vi "Generater.TestLauncher.vi"() -> ()   [LabVIEW 2019, in "Generator.lvclass"]
uses:
  Generator.lvclass
  typedefs/AO.Channel--Cluster--Array.ctl
  typedefs/AO.Channel--Cluster.ctl
  typedefs/AO.Channel.Function--Enum.ctl
  typedefs/REF.Channel--Cluster--Array.ctl
  typedefs/REF.Channel--Cluster.ctl
  typedefs/Sampling--Cluster.ctl
  typedefs/Sweep.Configuration--Cluster.ctl
  typedefs/Sweep.Channel--Cluster--Array.ctl
  typedefs/Sweep.Channel--Cluster.ctl
  typedefs/Sweep.Pattern--Enum.ctl
  typedefs/Generator.Command--enum.ctl
  typedefs/Generator.Sweep Status--enum.ctl
  <userlib>/LevyLab/Debug/Attribute.Debug/DebugBehavior.ctl
  C:/Program Files/National Instruments/LabVIEW 2019/vi.lib/JKI/JKI SMO/SMO/SMO.lvclass
  <vilib>/JKI/JKI SMO/SMO/SMO.lvclass/SMO.ctl
  <vilib>/JKI/JKI SMO/SMO/Typedefs/SMOState --Enum.ctl
  <vilib>/JKI/JKI SMO/SMO/Private/ReftoDVR--SMO.vi
  <vilib>/JKI/JKI SMO/SMO/SMO.lvclass
  <userlib>/LevyLab/Debug/Debug.lvlib
  <userlib>/LevyLab/Debug/Attribute.Debug/Attribute.Debug.lvclass
panel:
  in  "timeout":i32
  in  "Execute":bool
  out "sweep status":T1=enum."sweeping"
  out "Waveforms":waveform(dbl)[](graph)
  out "Waveform Chart":u32(graph)
  in  "command":T2=enum."stop"
  in  "Sweep Channels":T3 {"Channels"."Table" format="%#_1f"; "Channels"."Channel" min=1 max=128; "Channels"."Start" format="%#_6p"; "Channels"."End" format="%#_6p"}
  in  "Sampling":T7
  in  "REF Channels":T8
  in  "AO Channels":T10
  out "error out":errorcluster
  # "Close Panel to stop the SMO\n(press the \"X\")"
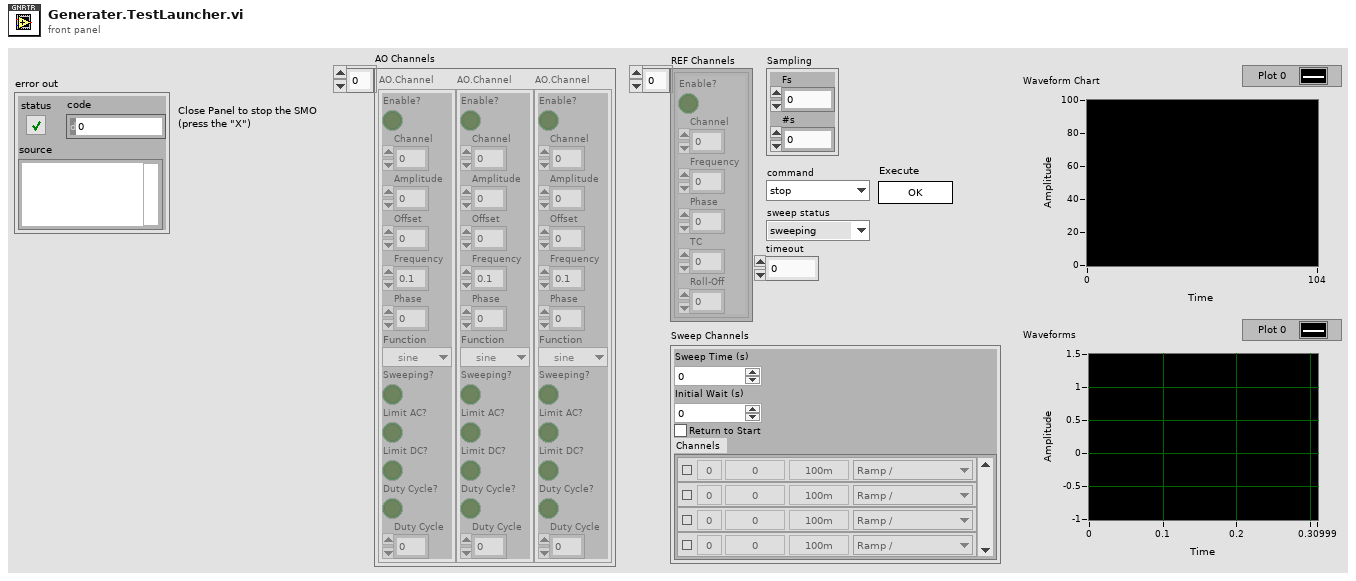
[diagram p1: front panel]
types:
  T1 = typedef "Generator.lvclass/Generator.Sweep Status--enum.ctl" = enum16{"idle", "initializing", "waiting", "sweeping", "stopping"}
  T2 = typedef "Generator.lvclass/Generator.Command--enum.ctl" = enum16{"start", "stop", "start sweep", "stop sweep"}
  T3 = typedef "Generator.lvclass/Sweep.Configuration--Cluster.ctl" = cluster{"Sweep Time (s)":dbl, "Initial Wait (s)":dbl, "Return to Start":bool, "Channels":T4}
  T4 = typedef "Generator.lvclass/Sweep.Channel--Cluster--Array.ctl" = T5[]
  T5 = typedef "Generator.lvclass/Sweep.Channel--Cluster.ctl" = cluster{"Enable?":bool, "Channel":u16, "Start":dbl, "End":dbl, "Pattern":T6, "Table":dbl[]}
  T6 = typedef "Generator.lvclass/Sweep.Pattern--Enum.ctl" = enum16{"Ramp /", "Ramp /\\", "Smooth Ramp _/", "Smooth Ramp _/\\_", "Table"}
  T7 = typedef "Generator.lvclass/Sampling--Cluster.ctl" = cluster{"Fs":dbl, "#s":dbl}
  T8 = typedef "Generator.lvclass/REF.Channel--Cluster--Array.ctl" = T9[]
  T9 = typedef "Generator.lvclass/REF.Channel--Cluster.ctl" = cluster{"Enable?":bool, "Channel":i32, "Frequency":dbl, "Phase":dbl, "TC":dbl, "Roll-Off":i32}
  T10 = typedef "Generator.lvclass/AO.Channel--Cluster--Array.ctl" = T11[]
  T11 = typedef "Generator.lvclass/AO.Channel--Cluster.ctl" = cluster{"Enable?":bool, "Channel":i32, "Amplitude":dbl, "Offset":dbl, "Frequency":dbl, "Phase":dbl, "Function":T12, "Sweeping?":bool, "Limit AC?":bool, "Limit DC?":bool, "Duty Cycle?":bool, "Duty Cycle":dbl}
  T12 = typedef "Generator.lvclass/AO.Channel.Function--Enum.ctl" = enum16{"sine", "square", "triangle", "saw"}
  T13 = typedef "Debug.lvlib/Attribute.Debug.lvclass/DebugBehavior.ctl" = enum16{"Normal", "Debug"}
  T14 = typedef "Generator.lvclass/PublicEvents--Cluster.ctl" = cluster{"Status":refnum<user-event>, "SweepStatus":refnum<user-event>, "AOChannels":refnum<user-event>, "Waveforms":refnum<user-event>}
  T15 = typedef "SMO.lvclass/Public Events.ctl" = cluster{"Error":refnum<user-event>, "State":refnum<user-event>, "Reserve State":refnum<user-event>}
  T16 = cluster{"Event Registration Refnum":refnum<event-registration>}
  T17 = typedef "SMO.lvclass/SMOState --Enum.ctl" = enum16{"unknown", "Created", "Started", "Stopped"}
  T18 = typedef "Generator.lvclass/Waveforms--Cluster.ctl" = cluster{"AO":waveform(dbl)[], "REF_X":waveform(dbl)[], "REF_Y":waveform(dbl)[]}
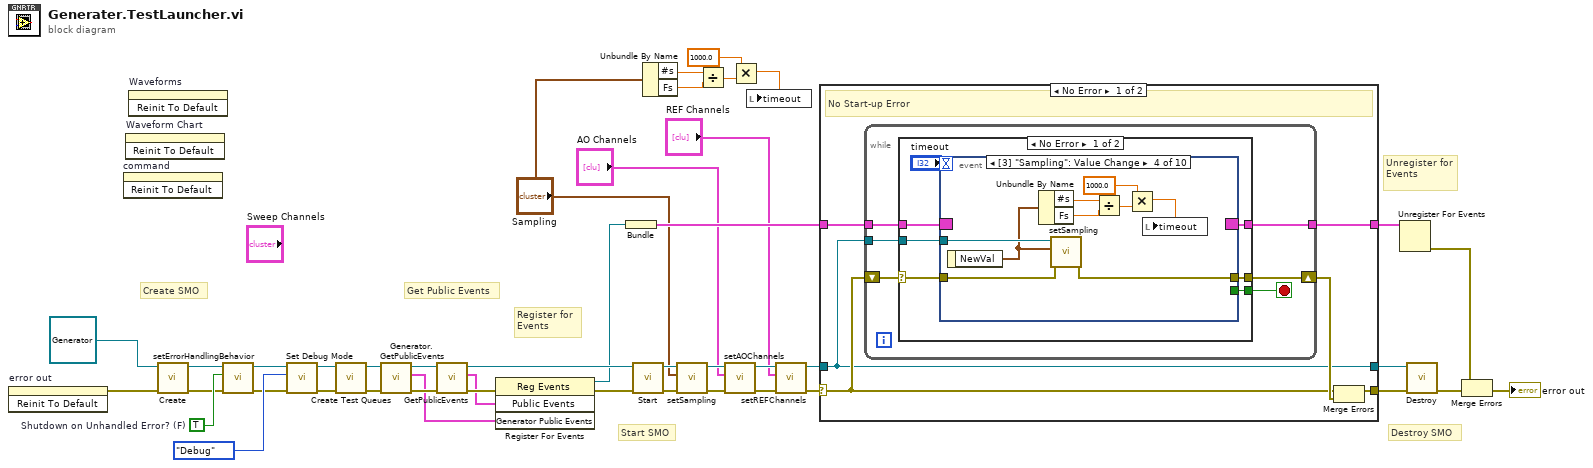
[diagram p0: block diagram]
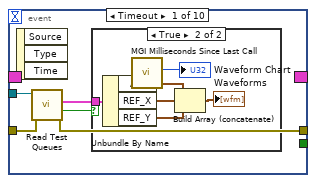
[diagram p2: hidden frame]
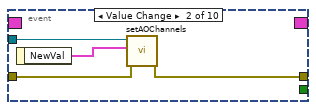
[diagram p4: hidden frame]
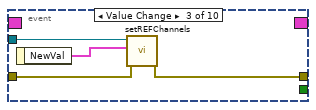
[diagram p5: hidden frame]
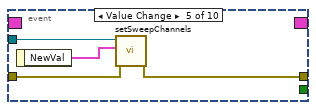
[diagram p6: hidden frame]
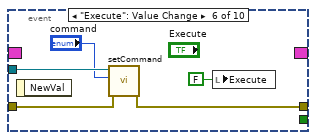
[diagram p7: hidden frame]
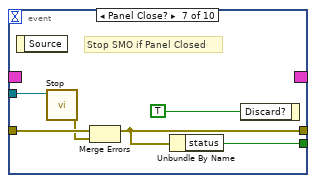
[diagram p8: hidden frame]
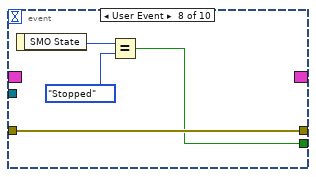
[diagram p9: hidden frame]
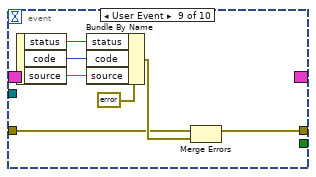
[diagram p10: hidden frame]
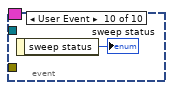
[diagram p11: hidden frame]
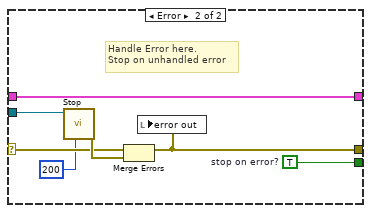
[diagram p12: hidden frame]
diagram:
  w40 = TRUE  # Shutdown on Unhandled Error? (F)
  # "Get Public Events"
  # "Start SMO"
  # "Destroy SMO"
  # "Create SMO"
  # "Unregister for Events"
  # "Register for Events"
  n1 = invoke on="error out" class="Clust (strict)" method="Reinit To Default"() -> (error out=w41:errorcluster)  [unwired: 3 in, 2 out]
  n2 = invoke on="command" class="Enum (strict)" method="Reinit To Default"() -> ()  [unwired: 3 in, 3 out]
  n3 = invoke on="Waveform Chart" class="WFChart (strict)" method="Reinit To Default"() -> ()  [unwired: 3 in, 3 out]
  n4 = invoke on="Waveforms" class="WFGraph (strict)" method="Reinit To Default"() -> ()  [unwired: 3 in, 3 out]
  n5 = call <vilib>:"Create.vi"("error in (no error)"=w41, "SMO"=refnum<class "Generator.lvclass"> refnum ("Generator.lvclass")) -> ("error out"=w39:errorcluster, "SMO out"=w38:refnum<class "Generator.lvclass">)  [unwired: 7 in, 1 out]
  n6 = call <vilib>:"setErrorHandlingBehavior.vi"("error in (no error)"=w39, "Shutdown on Unhandled Error? (F)"=w40, "SMO in"=w38) -> ("error out"=w24:errorcluster, "SMO out"=w25:refnum<class "Generator.lvclass">)  [unwired: 7 in]
  n7 = call <userlib>:"Set Debug Mode.vi"("error in (no error)"=w24, "Behavior"=DebugBehavior."Debug", "SMO"=w25) -> ("error out"=w11:errorcluster, "SMO out"=w23:refnum<class "Generator.lvclass">)  [unwired: 7 in]
  n8 = call "Create Test Queues.vi"("error in (no error)"=w11, "Generator in"=w23) -> ("error out"=w10:errorcluster, "Generator out"=w12:refnum<class "Generator.lvclass">)  [unwired: 8 in]
  n9 = call "Generator.GetPublicEvents.vi"("error in (no error)"=w10, "Generator"=w12) -> ("error out"=w9:errorcluster, "Generator Public Events"=w8:T14, "Generator out"=w7:refnum<class "Generator.lvclass">)  [unwired: 7 in]
  n10 = call <vilib>:"GetPublicEvents.vi"("error in (no error)"=w9, "SMO"=w7) -> ("error out"=w36:errorcluster, "Public Events"=w35:T15, "SMO out"=w42:refnum<class "Generator.lvclass">)  [unwired: 7 in]
  n11 = register-events(error in=w36, w35, w8) -> (reference out=w33:refnum<event-registration>, error out=w34:errorcluster)  [unwired: 1 in]
  n12 = Bundle("Event Registration Refnum"=w33) -> (w29:T16)  [unwired: 1 in]
  n13 = call <vilib>:"Start.vi"("error in (no error)"=w34, "SMO"=w42) -> ("error out"=w18:errorcluster, "SMO out"=w17:refnum<class "Generator.lvclass">)  [unwired: 8 in]
  n14 = Unbundle By Name("Sampling") -> ("#s"=w2:dbl, "Fs"=w3:dbl)
  n15 = call "setSampling.vi"("error in (no error)"=w18, "Sampling"="Sampling", "Generator in"=w17) -> ("error out"=w20:errorcluster, "Generator out"=w19:refnum<class "Generator.lvclass">)  [unwired: 7 in]
  n16 = Divide(x=w2, y=w3) -> (x/y=w4:dbl)
  n17 = call "setAOChannels.vi"("error in (no error)"=w20, "AO Channels"="AO Channels", "Generator in"=w19) -> ("error out"=w22:errorcluster, "Generator out"=w21:refnum<class "Generator.lvclass">)  [unwired: 7 in]
  n18 = Multiply(x=1000.0, y=w4) -> (x*y=w6:dbl)
  n19 = local write "timeout"(w6) -> ()
  n20 = call "setREFChannels.vi"("error in (no error)"=w22, "REF Channels"="REF Channels", "Generator in"=w21) -> ("error out"=w15:errorcluster, "Generator out"=w16:refnum<class "Generator.lvclass">)  [unwired: 7 in]
  n21 = case shown="No Error" w15 {
    selector: w15 -> [w45 w126]
    tunnel: [w49 w127] -> w28
    tunnel: w29 -> [w48 w127]
    tunnel: [w46 w126] -> w37
    tunnel: w16 -> [w44 w125]
    tunnel: [w44 w125] -> w43
    frame No Error {
      # "No Start-up Error"
      n22 = while {
        shift-right: [w54] -> w47
        shift-left: w45 -> [w50]
        tunnel: w48 -> [w53]
        tunnel: [w52] -> w49
        tunnel: w44 -> [w51]
        stop <- w55 stop-if-true
        n23 = case shown="No Error" w50 {
          selector: w50 -> [w57 w121]
          tunnel: [w62 w124] -> w55
          tunnel: [w61 w118] -> w54
          tunnel: w53 -> [w60 w123]
          tunnel: [w59 w123] -> w52
          tunnel: w51 -> [w58 w120]
          frame No Error {
            n24 = event shown="[3] \"Sampling\": Value Change" {
              selector: w60 -> [_ _ _ _ _ _ _ _ _ _]
              dyn-events: [_ _ _ _ _ _ _ _ _ _] -> w59
              timeout: "timeout" -> [_ _ _ _ _ _ _ _ _ _]
              tunnel: [_ _ _ _ _ _ w103 w106 _ _] -> w62
              tunnel: w58 -> [w67 w77 w79 w90 w94 w99 w105 _ _ _]
              tunnel: [w65 w74 w81 w88 w91 w97 w100 w107 w110 _] -> w61
              tunnel: w57 -> [w66 w75 w80 w89 w92 w98 w102 w107 w111 _]
              event Timeout {
                n25 = event-data() -> ()  [unwired: 1 in, 3 out]
                n26 = call "Read Test Queues.vi"("error in (no error)"=w66, "Generator in"=w67) -> ("error out"=w65:errorcluster, "result?"=w63:bool, "waveforms"=w64:T18)  [unwired: 6 in, 1 out]
                n27 = case shown="True" w63 {
                  tunnel: w64 -> [_ w73]
                  frame False {
                  }
                  frame True {
                    n28 = Unbundle By Name(w73) -> ("AO"=w71:waveform(dbl)[], "REF_X"=w68:waveform(dbl)[], "REF_Y"=w69:waveform(dbl)[])
                    n29 = call <userlib>:"MGI Milliseconds Since Last Call.vi"() -> ("ms"=→"Waveform Chart":u32)  [unwired: 6 in, 1 out]
                    n30 = Build Array (concatenate)(w71, w68, w69) -> (→"Waveforms":waveform(dbl)[])
                  }
                }
              }
              event Value Change {
                n31 = event-data() -> ("NewVal"=w76:T10)  [unwired: 1 in]
                n32 = call "setAOChannels.vi"("error in (no error)"=w75, "AO Channels"=w76, "Generator in"=w77) -> ("error out"=w74:errorcluster)  [unwired: 7 in, 1 out]
              }
              event Value Change {
                n33 = event-data() -> ("NewVal"=w78:T8)  [unwired: 1 in]
                n34 = call "setREFChannels.vi"("error in (no error)"=w80, "REF Channels"=w78, "Generator in"=w79) -> ("error out"=w81:errorcluster)  [unwired: 7 in, 1 out]
              }
              event Value Change {
                n35 = event-data() -> ("NewVal"=w87:T7)  [unwired: 1 in]
                n36 = Unbundle By Name(w87) -> ("#s"=w86:dbl, "Fs"=w85:dbl)
                n37 = call "setSampling.vi"("error in (no error)"=w89, "Sampling"=w87, "Generator in"=w90) -> ("error out"=w88:errorcluster)  [unwired: 7 in, 1 out]
                n38 = Divide(x=w86, y=w85) -> (x/y=w84:dbl)
                n39 = Multiply(x=1000.0, y=w84) -> (x*y=w82:dbl)
                n40 = local write "timeout"(w82) -> ()
              }
              event Value Change {
                n41 = event-data() -> ("NewVal"=w93:T3)  [unwired: 1 in]
                n42 = call "setSweepChannels.vi"("error in (no error)"=w92, "Sweep Channels"=w93, "Generator in"=w94) -> ("error out"=w91:errorcluster)  [unwired: 7 in, 1 out]
              }
              event "Execute": Value Change {
                n43 = event-data() -> ()  [unwired: 1 in, 1 out]
                n44 = call "setCommand.vi"("error in (no error)"=w98, "command"="command", "Generator in"=w99) -> ("error out"=w97:errorcluster)  [unwired: 7 in, 1 out]
                n45 = local write "Execute"(FALSE ("Execute")) -> ()
              }
              event Panel Close? {
                # "Stop SMO if Panel Closed"
                n46 = event-data() -> ()  [unwired: 1 in, 1 out]
                n47 = call <vilib>:"Stop.vi"("SMO"=w105) -> ("error out"=w101:errorcluster)  [unwired: 9 in, 1 out]
                n48 = Merge Errors(w102, w101) -> (w100:errorcluster)
                n49 = Unbundle By Name(w100) -> ("status"=w103:bool)
                n50 = event-data("Discard?"=TRUE ("OK")) -> ()  [unwired: 1 in, 1 out]
              }
              event User Event {
                n51 = event-data() -> ("SMO State"=w109:T17)  [unwired: 1 in]
                n52 = Equal?(x=w109, y=SMOState_--Enum."Stopped") -> (x = y?=w106:bool)
              }
              event User Event {
                n53 = event-data() -> ("status"=w116:bool, "code"=w115:i32, "source"=w114:string)  [unwired: 1 in]
                n54 = Bundle By Name(cluster=errorcluster {"status"=FALSE, "code"=0, "source"=""} ("error out"), "status"=w116, "code"=w115, "source"=w114) -> (w112:errorcluster)
                n55 = Merge Errors(w111, w112) -> (w110:errorcluster)
              }
              event User Event {
                n56 = event-data() -> ("sweep status"=→"sweep status":T1)  [unwired: 1 in]
              }
            }
          }
          frame Error {
            w124 = TRUE  # stop on error?
            # "Handle Error here.\nStop on unhandled error"
            n57 = call <vilib>:"Stop.vi"("timeout in ms (-1)"=200, "SMO"=w120) -> ("error out"=w122:errorcluster)  [unwired: 8 in, 1 out]
            n58 = Merge Errors(w121, w122) -> (w118:errorcluster)
            n59 = local write "error out"(w118) -> ()
          }
        }
      }
      n60 = Merge Errors(w45, w47) -> (w46:errorcluster)
    }
    frame Error {
      # "Error occured before starting the process"
    }
  }
  n61 = Unregister For Events(event registration refnum=w28) -> (error out=w30:errorcluster)  [unwired: 1 in]
  n62 = call <vilib>:"Destroy.vi"("error in (no error)"=w37, "SMO"=w43) -> ("error out"=w32:errorcluster)  [unwired: 9 in]
  n63 = Merge Errors(w30, w32) -> (→"error out":errorcluster)
